vi "Zero.vi"(0 "reference in":refnum<class "SmartMotor.lvclass">, 5 "error in (no error)":errorcluster) -> (14 "reference out":refnum<class "SmartMotor.lvclass">, 19 "error out":errorcluster)   [LabVIEW 2017]
uses:
  SmartMotor.lvclass
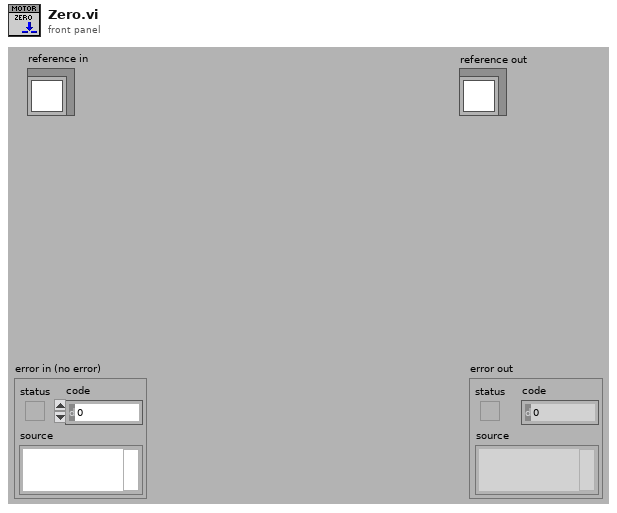
[diagram p1: front panel]
types:
  T1 = typedef "SmartMotor.lvclass/ObjectAttributes.ctl" = cluster{"Workstation Number":u8, "Motor Address Number":u8, "Motor Status":T2, "VISA resource name":refnum<visa-resource-name>}
  T2 = typedef "Motor Status.ctl" = enum8{"Off", "Initializing", "Stopped", "Rotating", "Fault"}
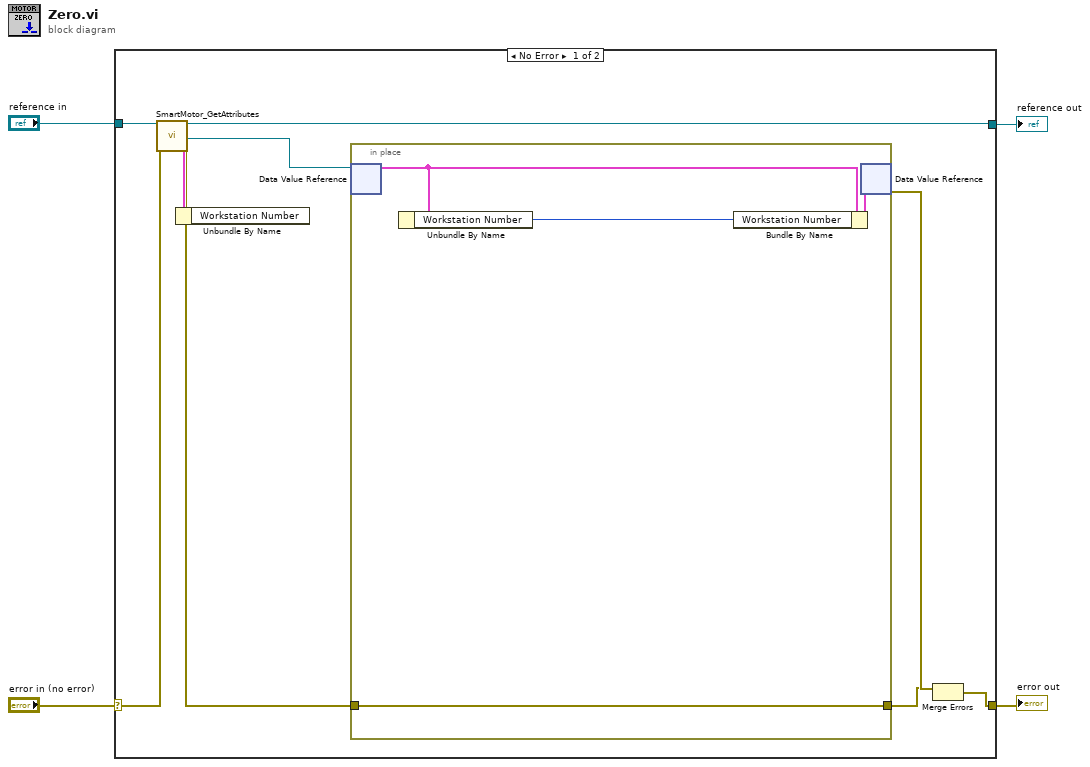
[diagram p0: block diagram]
diagram:
  n1 = case shown="No Error" "error in (no error)" {
    selector: "error in (no error)" -> [w12 w19]
    tunnel: [w8 w19] -> w3
    tunnel: [w9 w18] -> w1
    tunnel: "reference in" -> [w13 w18]
    frame No Error {
      n2 = call "SmartMotor_GetAttributes.vi"("reference in"=w13, "error in (no error)"=w12) -> ("reference out"=w9:refnum<class "SmartMotor.lvclass">, "Data"=w11:T1, "DataRef"=w7:refnum<data-value>, "error out"=w6:errorcluster)  [unwired: 14 in]
      n3 = Unbundle By Name(w11) -> ()  [unwired: 1 out]
      n4 = in-place {
        in-place-border: w6 -> [w14]
        in-place-border: [w14] -> w5
        n5 = in-place-dvr #1(w7) -> (w16:T1)  [unwired: 1 out]
        n6 = Unbundle By Name(w16) -> ("Workstation Number"=w15:u8)
        n7 = Bundle By Name(cluster=w16, "Workstation Number"=w15) -> (w17:T1)
        n8 = in-place-dvr #1(w17) -> (w10:errorcluster)  [unwired: 1 out]
      }
      n9 = Merge Errors(w10, w5) -> (w8:errorcluster)
    }
    frame Error {
    }
  }
  "error out" <- w3
  "reference out" <- w1
